vi "Split Flattened Strings.vi"(11 "Flattened Strings":string) -> (3 "Strings":string[](array[string]))   [LabVIEW 2021, in "BS120x Driver.lvlib"]
uses:
  BS120x Driver.lvlib
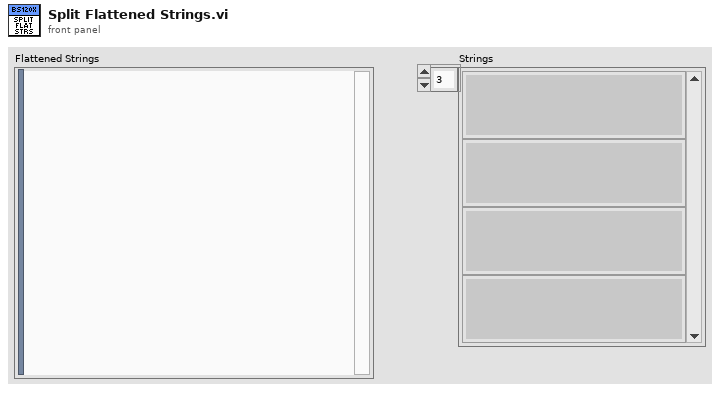
[diagram p1: front panel]
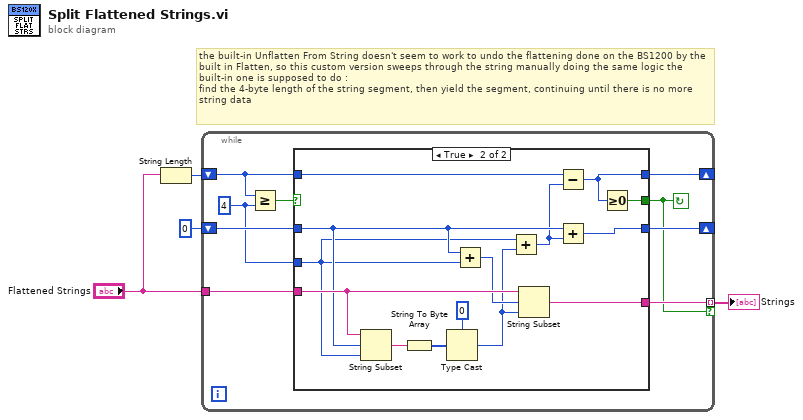
[diagram p0: block diagram]
diagram:
  # "the built-in Unflatten From String doesn't seem to work to undo the flattening done on the BS1200 by the built in Flatten, so this custom version sweeps through the string manually doing the same logic the built-in one is supposed to do :\nfind the 4-byte length of the string segment, then yield the segment, continuing until there is no more string data"
  n1 = String Length(string="Flattened Strings") -> (length=w1:i32)
  n2 = while {
    tunnel: "Flattened Strings" -> [w13]
    shift-right: [w11] -> _
    shift-left: 0 -> [w12]
    tunnel: [w10] -> w4 mode=indexing if=w5
    shift-right: [w6] -> _
    shift-left: w1 -> [w7]
    stop <- w5 continue-if-true
    w9 = 4 ("y")
    n3 = Greater Or Equal?(x=w7, y=w9) -> (x >= y?=w8:bool)
    n4 = case shown="True" w8 {
      selector: w8 -> [w15 _]
      tunnel: w13 -> [_ w27]
      tunnel: w12 -> [w14 w26]
      tunnel: [w14 w24] -> w11
      tunnel: [_ w23] -> w10
      tunnel: w9 -> [_ w21]
      tunnel: w7 -> [w16 w20]
      tunnel: [w16 w18] -> w6
      tunnel: [w15 w17] -> w5
      frame False {
      }
      frame True {
        n5 = String Subset(string=w27, offset (0)=w26, length (rest)=w21) -> (substring=w30:string)
        n6 = String To Byte Array(string=w30) -> (unsigned byte array=w29:u8[])
        n7 = Type Cast(type=0, x=w29) -> (*(type *) &x=w22:i32)
        n8 = Add(x=w26, y=w21) -> (x+y=w25:i32)
        n9 = Add(x=w21, y=w22) -> (x+y=w19:i32)
        n10 = String Subset(string=w27, offset (0)=w25, length (rest)=w22) -> (substring=w23:string)
        n11 = Subtract(x=w20, y=w19) -> (x-y=w18:i32)
        n12 = Add(x=w26, y=w19) -> (x+y=w24:i32)
        n13 = Greater Or Equal To 0?(x=w18) -> (x >= 0?=w17:bool)
      }
    }
  }
  "Strings" <- w4
